vi "Enable_Baxter.vi"(0 "error in":errorcluster, 2 "Enable?":bool=TRUE, 3 "node":string) -> (1 "error out":errorcluster)   [LabVIEW 2013]
doc: "This will enable all the motors on Baxter"
uses:
  ROS/MessageBuilding/Primitives/subs/boolScalar.vi
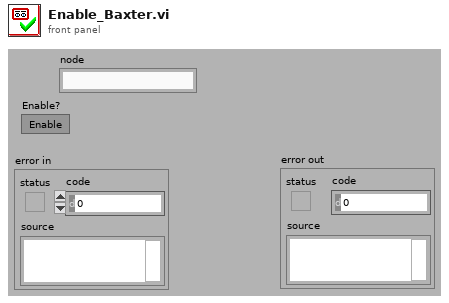
[diagram p1: front panel]
types:
  T1 = typedef "_ROSControl.ctl" = cluster{"topic port":u16, "Node":string, "topic":string, "type":string, "node port":u32, "error ":errorcluster, "Direction":T2, "APIs":string[]}
  T2 = typedef "_ROSDirection.ctl" = enum16{"Node", "Publisher", "Subscriber", "Service Client"}
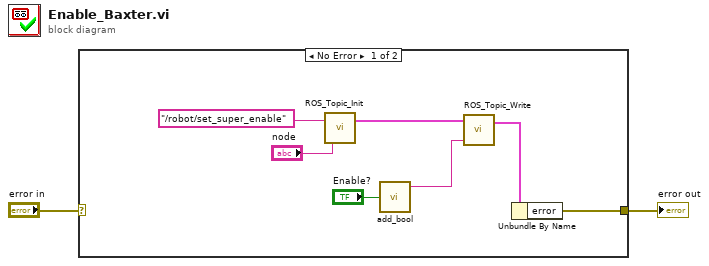
[diagram p0: block diagram]
diagram:
  n1 = case shown="No Error" "error in" {
    selector: "error in" -> [_ w10]
    tunnel: [w6 w10] -> w2
    frame No Error {
      n2 = call "ROS_Topic_Init.vi"("node"="node", "topic"="/robot/set_super_enable") -> ("ROS out"=w8:T1)  [unwired: 1 in]
      n3 = call-poly "add_bool.vi"("Boolean"="Enable?") -> ("msg out"=w4:string)  [unwired: 4 in]
      n4 = call "ROS_Topic_Write.vi"("Msg in"=w4, "ROS in"=w8) -> ("ROS out"=w7:T1)  [unwired: 2 in]
      n5 = Unbundle By Name(w7) -> ("error"=w6:errorcluster)
    }
    frame Error {
    }
  }
  "error out" <- w2
